vi "LVProjectShortcut_OnShortcutEdit.vi"(6 "error in":errorcluster, 9 "Wizard":T1) -> (0 "error out":errorcluster)   [LabVIEW 2017]
doc: "Use this template to create a wizard dialog."
uses:
  <resource>/Framework/Providers/API/ItemRef.ctl
  <resource>/Framework/Providers/API/mxLvChangeType.ctl
panel:
  in  "Cancel":bool
  in  "OK":bool
  in  "File Path":path caption="Target"
  in  "Name":string caption="Shortcut name"
  # "Shortcut edition"
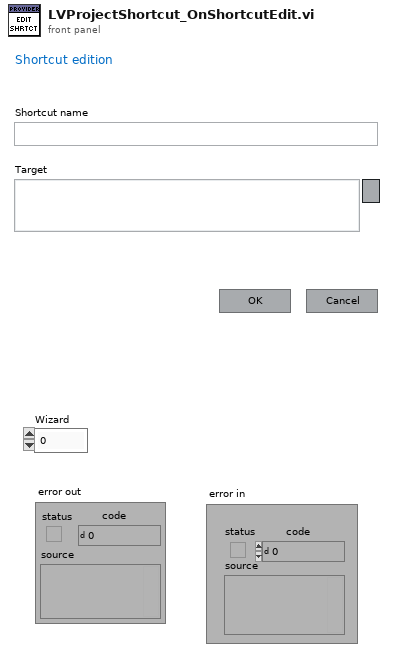
[diagram p1: front panel]
types:
  T1 = typedef "ItemRef.ctl" = u64
  T2 = typedef "mxLvChangeType.ctl" = enum32{"Item Created", "Item Modified", "File Modified", "File Deleted", "Item Added", "Item Added to SCC", "Item Renamed", "Item Modified For SCC"}
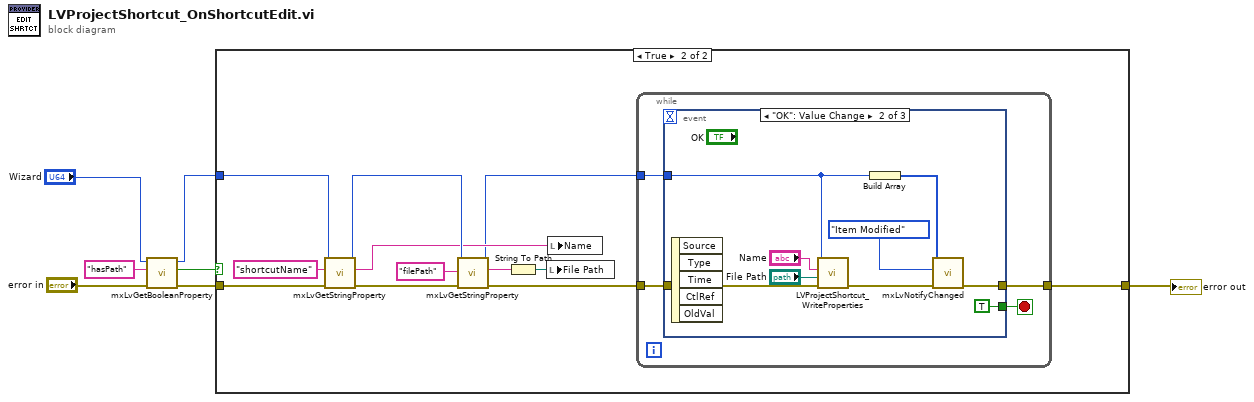
[diagram p0: block diagram]
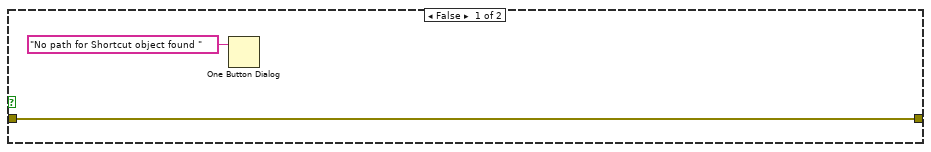
[diagram p2: hidden frame]
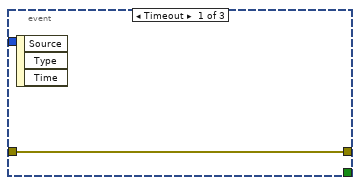
[diagram p3: hidden frame]
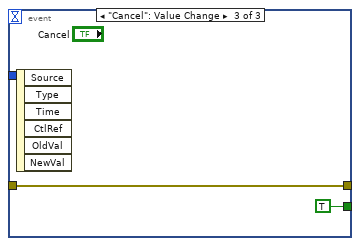
[diagram p4: hidden frame]
diagram:
  n1 = call <resource>:"mxLvGetBooleanProperty.vi"("error in"="error in", "Tag"="hasPath", "Item"="Wizard") -> ("error out"=w6:errorcluster, "Value"=w5:bool, "Item"=w4:T1)  [unwired: 6 in]
  n2 = case shown="True" w5 {
    tunnel: w4 -> [_ w13]
    tunnel: w6 -> [w9 w21]
    tunnel: [w9 w11] -> w1
    frame False {
      n3 = One Button Dialog(message="No path for Shortcut object found ") -> ()  [unwired: 1 in, 1 out]
    }
    frame True {
      n4 = call <resource>:"mxLvGetStringProperty.vi"("Error In"=w21, "Tag"="shortcutName", "Item"=w13) -> ("Error Out"=w20:errorcluster, "Value"=w16:string, "Item"=w17:T1)  [unwired: 6 in]
      n5 = call <resource>:"mxLvGetStringProperty.vi"("Error In"=w20, "Tag"="filePath", "Item"=w17) -> ("Error Out"=w12:errorcluster, "Value"=w15:string, "Item"=w10:T1)  [unwired: 6 in]
      n6 = String To Path(string=w15) -> (path=w14:path)
      n7 = local write "File Path"(w14) -> ()
      n8 = local write "Name"(w16) -> ()
      n9 = while {
        tunnel: w12 -> [w25]
        tunnel: [w24] -> w11
        tunnel: w10 -> [w22]
        stop <- w23 stop-if-true
        n10 = event shown="[1] \"OK\": Value Change" {
          selector: _ -> [_ _ _]
          dyn-events: _ -> [_ _ _]
          timeout: _ -> [_ _ _]
          tunnel: w25 -> [w26 w35 w37]
          tunnel: [w26 w27 w37] -> w24
          tunnel: [_ TRUE TRUE] -> w23
          tunnel: w22 -> [_ w29 _]
          event Timeout {
            n11 = event-data() -> ()  [unwired: 1 in, 3 out]
          }
          event "OK": Value Change {
            n12 = event-data() -> ()  [unwired: 1 in, 5 out]
            n13 = call <resource>:"LVProjectShortcut_WriteProperties.vi"("error in"=w35, "filePath"="File Path", "shortcutName"="Name", "Wizard"=w29) -> ("error out"=w28:errorcluster)  [unwired: 7 in]
            n14 = Build Array(w29) -> (w31:T1[])
            n15 = call <resource>:"mxLvNotifyChanged.vi"("error in (no error)"=w28, "Change Type"=mxLvChangeType."Item Modified", "Items"=w31) -> ("error out"=w27:errorcluster)  [unwired: 7 in, 1 out]
          }
          event "Cancel": Value Change {
            n16 = event-data() -> ()  [unwired: 1 in, 6 out]
          }
        }
      }
    }
  }
  "error out" <- w1
